vi "Write Format string.vi"(8 "error in (no error)":errorcluster, 10 "Format string":string, 11 "Floating point base in":refnum<class "Floating point base.lvclass">) -> (0 "error out":errorcluster, 3 "Floating point base out":refnum<class "Floating point base.lvclass">)   [LabVIEW 2018, in "D Datagrid Library.lvlib" / "Floating point base.lvclass"]
uses:
  Floating point base.lvclass
  Floating point base.lvclass/Floating point base.ctl
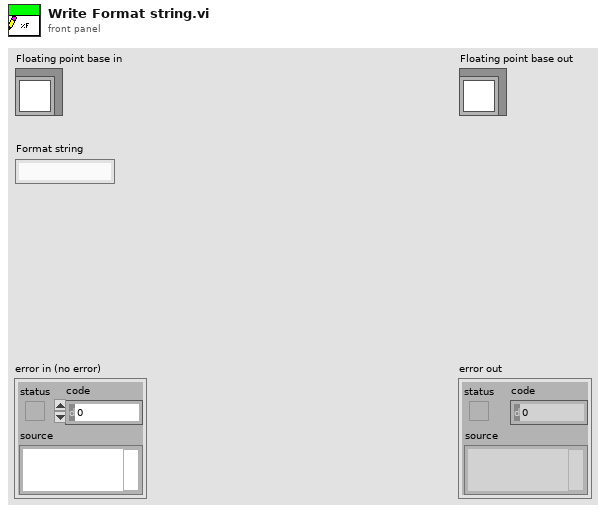
[diagram p1: front panel]
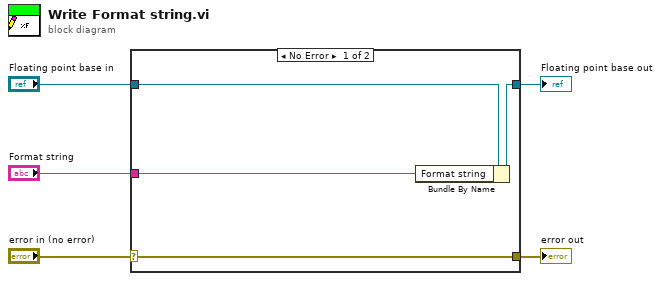
[diagram p0: block diagram]
diagram:
  n1 = case shown="No Error" "error in (no error)" {
    selector: "error in (no error)" -> [w9 w10]
    tunnel: [w9 w10] -> w4
    tunnel: [w7 w11] -> w2
    tunnel: "Floating point base in" -> [w8 w11]
    tunnel: "Format string" -> [w6 _]
    frame No Error {
      n2 = Bundle By Name(cluster=w8, "Format string"=w6) -> (w7:refnum<class "Floating point base.lvclass">)
    }
    frame Error {
    }
  }
  "error out" <- w4
  "Floating point base out" <- w2
